vi "Element Factory.vi"(8 "error in (no error)":errorcluster, 10 "Element":refnum<class "Config Element.lvclass">) -> (0 "error out":errorcluster, 3 "VCfg Element":refnum<class "VolatusConfigElement.lvclass">)   [LabVIEW 2020, in "VolatusConfig.lvlib"]
uses:
  VolatusConfig.lvlib
  lv-cdm/CDM-Config/Config Element/Config Element.lvclass
  Meta Name.ctl
  Meta Type.ctl
  System/System Config.lvclass
  VolatusConfigElement/VolatusConfigElement.lvclass
  C:/dev/lv20CE/relink/lv-volatus/VolatusConfig/VolatusConfigElement/VolatusConfigElement.lvclass
  C:/dev/lv20CE/relink/lv-volatus/VolatusConfig/System/System Config.lvclass
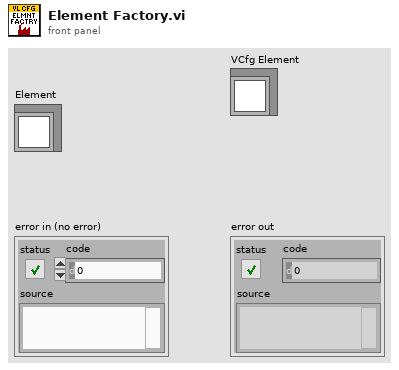
[diagram p1: front panel]
types:
  T1 = typedef "VolatusConfig.lvlib/Meta Type.ctl" = enum16{"UNKNOWN", "VL_System", "VL_Cluster", "VL_Node", "VL_Task", "VL_Group", "VL_Channel", "VL_Task_List", "VL_Scaling", "VL_Sensor", "VL_Sensor_List", "VL_Scale"}
  T2 = typedef "VolatusConfig.lvlib/Meta Name.ctl" = enum16{"VL_Type", "VL_Node_IP", "VL_Node_Type", "VL_Task_Type", "VL_Group_Type", "VL_Channel_Type", "VL_Channel_DataType", "VL_Config_Version", "VL_Overlay_Type", "VL_Config_Hash"}
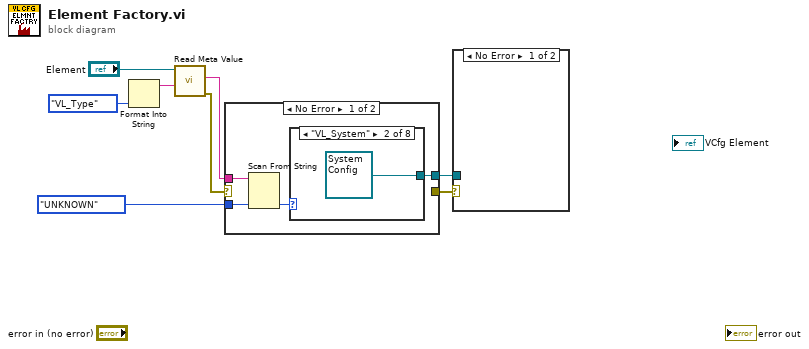
[diagram p0: block diagram]
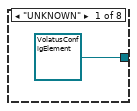
[diagram p2: hidden frame]
diagram:
  n1 = Format Into String(Meta_Name."VL_Type" ("Meta Name")) -> (resulting string=w6:string)  [unwired: 3 in, 1 out]
  n2 = call "Read Meta Value.vi"("Meta Name"=w6, "Config Element in"="Element") -> ("error out"=w3:errorcluster, "Meta Value"=w5:string)  [unwired: 7 in, 1 out]
  n3 = case shown="No Error" w3 {
    selector: w3 -> [_ w15]
    tunnel: w5 -> [w12 _]
    tunnel: Meta_Type."UNKNOWN" ("Meta Type") -> [w11 _]
    tunnel: [_ w15] -> w2
    tunnel: [w9 _] -> w1
    frame No Error {
      n4 = Scan From String(input string=w12, default 1=w11) -> (output 1=w10:T1)  [unwired: 3 in, 3 out]
      n5 = case shown="\"VL_System\"" w10 {
        tunnel: [refnum<class "VolatusConfigElement.lvclass"> refnum ("VolatusConfig.lvlib:VolatusConfigElement") refnum<class "System Config.lvclass"> refnum ("VolatusConfig.lvlib:System.lvclass") _ _ _ _ _ _] -> w9
        frame "UNKNOWN" {
        }
        frame "VL_System" {
        }
        frame "VL_Cluster" {
        }
        frame "VL_Node" {
        }
        frame "VL_Task" {
        }
        frame "VL_Group" {
        }
        frame "VL_Channel" {
        }
        frame "VL_Task_List" {
        }
      }
    }
    frame Error {
    }
  }
  n6 = case shown="No Error" w2 {
    tunnel: w1 -> [_ _]
    frame No Error {
    }
    frame Error {
    }
  }
